vi "Teleop.vi"(10 "Match Info":T1={"Autonomous Elapsed Seconds"=0.0, "TeleOp Elapsed Seconds"=0.0, "Disabled Elapsed Seconds"=0.0, "Visited Autonomous"=FALSE, "Visited TeleOp"=FALSE, "Visited Disabled"=FALSE, "Autonomous Settings"={"Autonomous Style"=enum."Independent", "VI Refnum"=refnum}}, 11 "Call Context":T2) -> ()   [LabVIEW 2018]
doc: "This VI is called for each enabled TeleOp packet received from the DS. It is typically used to read from joysticks and other inputs and update I/O or setpoints for timed control loops. It should complete and return within 20 milliseconds or risk missing DS packets."
uses:
  <vilib>/Rock Robotics/WPI/DriverStation/WPI_DriverStationDerivedRobotMode.ctl
  <vilib>/Rock Robotics/WPI/DriverStation/WPI_DriverStationMatch Info.ctl
  <vilib>/Rock Robotics/WPI/Utilities/WPI_GetSetVariantRefNum.vi
  <vilib>/Rock Robotics/Network Tables/NT Write Boolean Array.vi
  <vilib>/Rock Robotics/Network Tables/NT Write Numeric Array.vi
panel:
  in  "drive type":dbl=1.0 min=1.0 max=3.0 step=1.0
  # "1 for arcade,\n2 for tank,\n3 for cheesy"
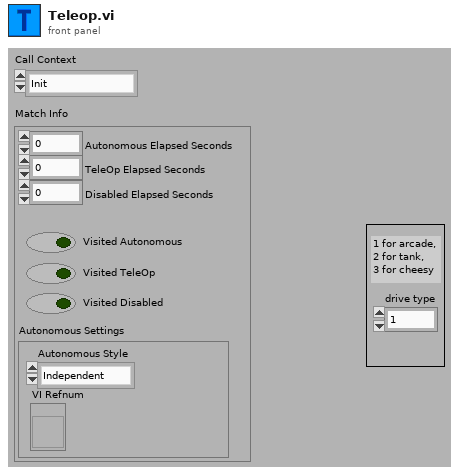
[diagram p1: front panel]
types:
  T1 = typedef "WPI_DriverStationMatch Info.ctl" = cluster{"Autonomous Elapsed Seconds":dbl, "TeleOp Elapsed Seconds":dbl, "Disabled Elapsed Seconds":dbl, "Visited Autonomous":bool, "Visited TeleOp":bool, "Visited Disabled":bool, "Autonomous Settings":cluster{"Autonomous Style":enum16{"Iterative", "Independent"}, "VI Refnum":refnum<vi>}}
  T2 = typedef "WPI_DriverStationDerivedRobotMode.ctl" = enum16{"Init", "Execute", "Stop"}
  T3 = typedef "WPI_JoystickDevRef.ctl" = cluster{"Device":T4}
  T4 = typedef "WPI_JoystickDeviceEnum.ctl" = enum16{"USB 0", "USB 1", "USB 2", "USB 3", "USB 4", "USB 5"}
  T5 = typedef "Command Status Info.ctl" = cluster{"Name":string, "Status":T6, "notifier out":T7}
  T6 = typedef "Completion Status.ctl" = enum16{"Successful", "Aborted", "Incomplete"}
  T7 = typedef "Completion Notifier.ctl" = refnum<notifier>
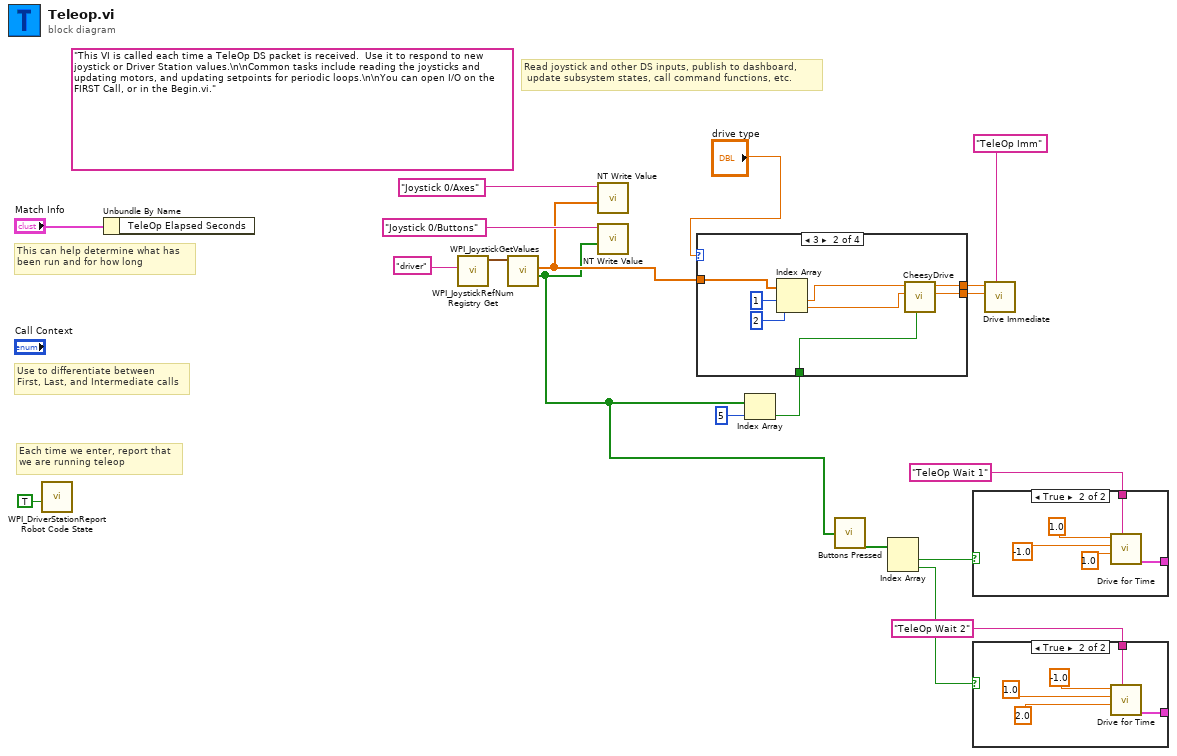
[diagram p0: block diagram]
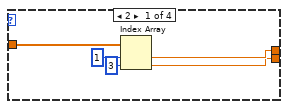
[diagram p2: hidden frame]
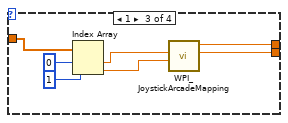
[diagram p3: hidden frame]
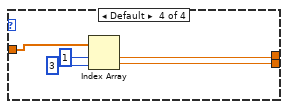
[diagram p4: hidden frame]
diagram:
  (unwired) "This VI is called each time a TeleOp DS packet is received.  Use it to respond to new joystick or Driver Station values.\n\nCommon tasks include reading the joysticks and updating motors, and updating setpoints for periodic loops.\n\nYou can open I/O on the FIRST Call, or in the Begin.vi."
  # "Read joystick and other DS inputs, publish to dashboard,\n update subsystem states, call command functions, etc."
  # "Each time we enter, report that\nwe are running teleop"
  # "Use to differentiate between\nFirst, Last, and Intermediate calls"
  # "This can help determine what has\nbeen run and for how long"
  n1 = call <vilib>:"WPI_DriverStationReport Robot Code State.vi"("TeleOp"=TRUE ("Autonomous")) -> ()  [unwired: 10 in, 1 out]
  n2 = Unbundle By Name("Match Info") -> ()  [unwired: 1 out]
  n3 = call <vilib>:"WPI_JoystickRefNum Registry Get.vi"("refnum name"="driver") -> ("JoystickDevRef"=w11:T3)  [unwired: 1 in, 9 out]
  n4 = call <vilib>:"WPI_JoystickGetValues.vi"("JoystickDevRef"=w11) -> ("Buttons"=w2:bool[], "Axes"=w5:dbl[])  [unwired: 6 in, 3 out]
  n5 = call-poly <vilib>:"NT Write Value.vi"("Numeric Array"=w5, "Name"="Joystick 0/Axes") -> ()  [unwired: 9 in, 1 out]
  n6 = call-poly <vilib>:"NT Write Value.vi"("Boolean Array"=w2, "Name"="Joystick 0/Buttons") -> ()  [unwired: 9 in, 1 out]
  n7 = Index Array(array=w2, index=5) -> (element=w4:bool)
  n8 = case shown="3" "drive type" {
    tunnel: [w21 w30 w39 w41] -> w9
    tunnel: [w20 w31 w38 w40] -> w8
    tunnel: w5 -> [w24 w32 w37 w44]
    tunnel: w4 -> [_ w27 _ _]
    frame 2 {
      n9 = Index Array(array=w24, index #1=1 ("index"), index #2=3 ("index")) -> (element #1=w21:dbl, element #2=w20:dbl)
    }
    frame 3 {
      n10 = Index Array(array=w32, index #1=1 ("index"), index #2=2 ("index")) -> (element #1=w26:dbl, element #2=w25:dbl)
      n11 = call "CheesyDrive.vi"("Quickturn"=w27, "Wheel"=w25, "Throttle"=w26) -> ("Right PWM"=w31:dbl, "Left PWM"=w30:dbl)  [unwired: 7 in]
    }
    frame 1 {
      n12 = Index Array(array=w37, index #1=0 ("index"), index #2=1 ("index")) -> (element #1=w36:dbl, element #2=w35:dbl)
      n13 = call <vilib>:"WPI_JoystickArcadeMapping.vi"("Y axis value"=w35, "X axis value"=w36) -> ("Right Motor Value"=w38:dbl, "Left Motor Value"=w39:dbl)  [unwired: 8 in]
    }
    frame Default {
      n14 = Index Array(array=w44, index #1=1 ("index"), index #2=3 ("index")) -> (element #1=w41:dbl, element #2=w40:dbl)
    }
  }
  n15 = call "Buttons Pressed.vi"("Button Values"=w2) -> ("Button Presses"=w15:bool[])
  n16 = Index Array(array=w15) -> (element #1=w14:bool, element #2=w13:bool)  [unwired: 2 in]
  n17 = case shown="True" w14 {
    tunnel: [_ w48] -> _
    tunnel: "TeleOp Wait 1" ("Description") -> [_ w47]
    frame False {
    }
    frame True {
      n18 = call "Drive for Time.vi"("Description"=w47, "Seconds"=1.0, "Right Speed"=-1.0, "Left Speed"=1.0) -> ("Command Info Out"=w48:T5)  [unwired: 7 in]
    }
  }
  n19 = case shown="True" w13 {
    tunnel: [_ w52] -> _
    tunnel: "TeleOp Wait 2" ("Description") -> [_ w51]
    frame False {
    }
    frame True {
      n20 = call "Drive for Time.vi"("Description"=w51, "Seconds"=2.0, "Right Speed"=1.0, "Left Speed"=-1.0) -> ("Command Info Out"=w52:T5)  [unwired: 7 in]
    }
  }
  n21 = call "Drive Immediate.vi"("Description"="TeleOp Imm", "Right Setpoint"=w8, "Left Setpoint"=w9) -> ()  [unwired: 8 in, 1 out]
